vi "BRig_dataCurrent_nTrial.vi"() -> (2 "output_nTrial":i32)   [LabVIEW 2014]
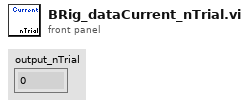
[diagram p1: front panel]
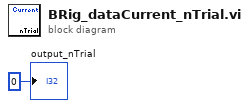
[diagram p0: block diagram]
diagram:
  "output_nTrial" <- 0 ("output_iBlock")
